vi "GOOP_StartDebuggerController.vi"(5 "error in (no error)":errorcluster) -> (19 "error out":errorcluster)   [LabVIEW 2016]
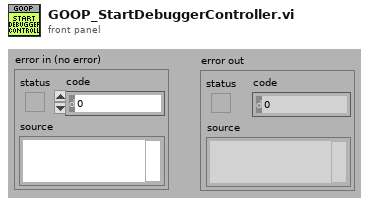
[diagram p1: front panel]
types:
  T1 = enum32{"Bad", "Idle", "Run top level", "Running"}
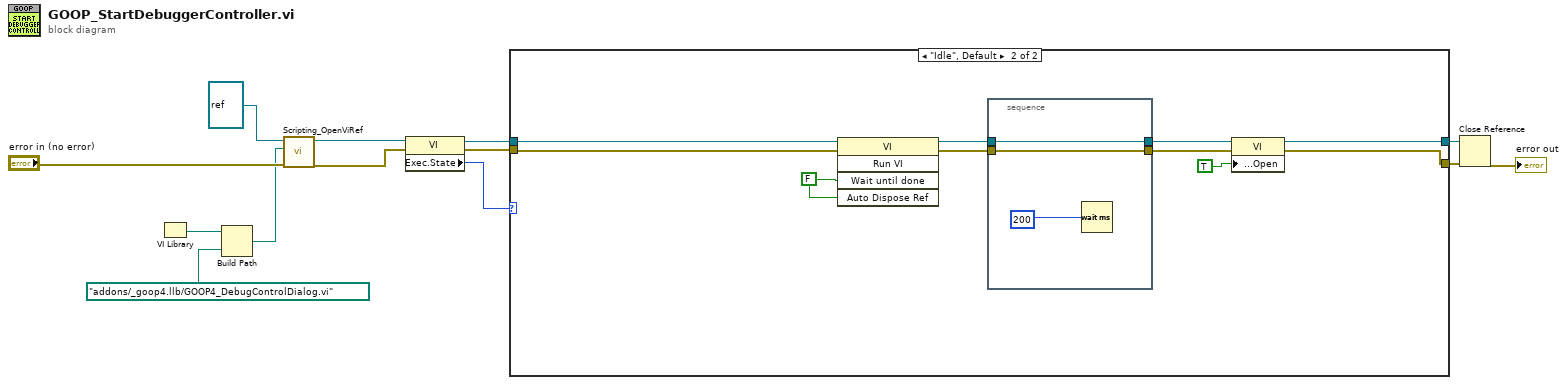
[diagram p0: block diagram]
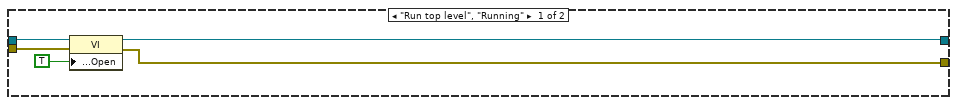
[diagram p2: hidden frame]
diagram:
  n1 = VI Library() -> (path=w2:path)
  n2 = Build Path(base path=w2, name or relative path=path "addons/_goop4.llb/GOOP4_DebugControlDialog.vi" ("base path")) -> (appended path=w10:path)
  n3 = call <resource>:"Scripting_OpenViRef.vi"("error in"="error in (no error)", "ViPath/ViName/Viref"=w10, "AppRef"=refnum<vi> refnum) -> ("error out"=w8:errorcluster, "vi reference"=w7:refnum<vi>)  [unwired: 6 in, 1 out]
  n4 = property class="VI"(reference=w7, error in=w8) -> (reference out=w5:refnum<vi>, error out=w6:errorcluster, "Exec.State"=w4:T1)
  n5 = case shown="\"Idle\", Default" w4 {
    tunnel: [w14 w23] -> w13
    tunnel: [w15 w24] -> w12
    tunnel: w6 -> [w17 w20]
    tunnel: w5 -> [w18 w19]
    frame "Run top level", "Running" {
      n6 = property class="VI"(reference=w18, error in=w17, "Front Panel.Open"=TRUE ("Front Panel Window:Open")) -> (reference out=w15:refnum<vi>, error out=w14:errorcluster)
    }
    frame "Idle", Default {
      w26 = FALSE ("Wait Until Done")
      n7 = invoke class="VI" method="Run VI"(reference=w19, error in=w20, "Wait until done"=w26, "Auto Dispose Ref"=w26) -> (reference out=w28:refnum<vi>, error out=w27:errorcluster)  [unwired: 1 in, 3 out]
      n8 = stacked-sequence {
        tunnel: w27 -> [w30]
        tunnel: w28 -> [w31]
        tunnel: [w31] -> w21
        tunnel: [w30] -> w22
        frame #0 {
          n9 = Wait (ms)(milliseconds to wait=200) -> ()  [unwired: 1 out]
        }
      }
      n10 = property class="VI"(reference=w21, error in=w22, "Front Panel.Open"=TRUE ("Front Panel Window:Open")) -> (reference out=w24:refnum<vi>, error out=w23:errorcluster)
    }
  }
  n11 = Close Reference(reference=w12, error in (no error)=w13) -> (error out=→"error out":errorcluster)
